vi "IMAQdx Configure Grab.vi"(8 "error in":errorcluster, 10 "Number of Buffers":u32=5, 11 "Session In":T1) -> (0 "error out":errorcluster, 3 "Session Out":T1)   [LabVIEW 2020, in "NI_Vision_Acquisition_Software.lvlib"]
doc: "Configures and starts a grab acquisition. A grab performs an acquisition that loops continually on a ring of buffers. Use the grab VI for high-speed image acquisition. Use the IMAQdx Grab VI to copy an image out of the buffer. If you call this VI before calling the IMAQdx Open Camera VI, the IMAQdx Configure Grab VI uses cam0 by default. Use the IMAQdx Unconfigure Acquisition VI to unconfigure the acquisition."
uses:
  NI_Vision_Acquisition_Software.lvlib
  IMAQdx.ctl
  IMAQdx Acquisition Mode.ctl
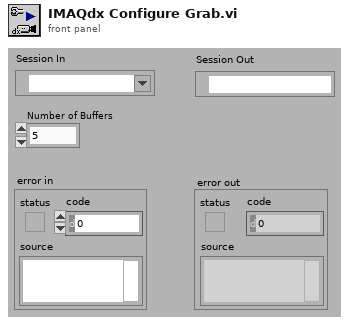
[diagram p1: front panel]
types:
  T1 = typedef "IMAQdx.ctl" = refnum<k21>
  T2 = typedef "NI_Vision_Acquisition_Software.lvlib/IMAQdx Acquisition Mode.ctl" = enum32{"One Shot", "Continuous"}
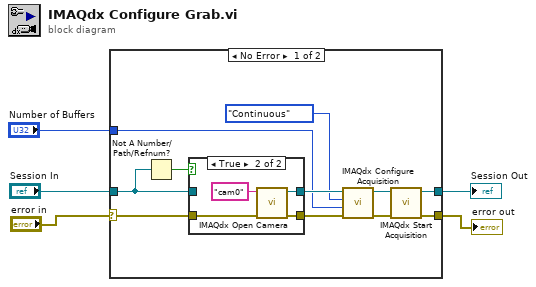
[diagram p0: block diagram]
diagram:
  n1 = case shown="No Error" "error in" {
    selector: "error in" -> [w7 w24]
    tunnel: "Session In" -> [w15 w23]
    tunnel: [w9 w23] -> w4
    tunnel: [w8 w24] -> w3
    tunnel: "Number of Buffers" -> [w6 _]
    frame No Error {
      n2 = Not A Number/Path/Refnum?(number/path/refnum=w15) -> (NaN/Path/Refnum?=w10:bool)
      n3 = case shown="True" w10 {
        tunnel: [w18 w22] -> w16
        tunnel: w15 -> [w18 _]
        tunnel: [w17 w21] -> w14
        tunnel: w7 -> [w17 w20]
        frame False {
        }
        frame True {
          n4 = call "IMAQdx Open Camera.vi"("error in"=w20, "Session In"="cam0") -> ("error out"=w21:errorcluster, "Session Out"=w22:T1)  [unwired: 8 in]
        }
      }
      n5 = call "IMAQdx Configure Acquisition.vi"("error in"=w14, "Number of Buffers"=w6, "Continuous?"=IMAQdx_Acquisition_Mode."Continuous", "Session In"=w16) -> ("error out"=w11:errorcluster, "Session Out"=w12:T1)  [unwired: 6 in]
      n6 = call "IMAQdx Start Acquisition.vi"("error in"=w11, "Session In"=w12) -> ("error out"=w8:errorcluster, "Session Out"=w9:T1)  [unwired: 8 in]
    }
    frame Error {
    }
  }
  "Session Out" <- w4
  "error out" <- w3
